vi "GeneratePSF.vi"(7 "Trans Geometry":T1={"Radius (cm)"=1.2, "a (cm)"=0.3, "focus location"=1.2} {"focus location" format="%.2f"; "a (cm)" format="%.2f"; "Radius (cm)" format="%.2f"}, 8 "Variables":T3={"Number of rings"=1, "sound spd (cm/s)"=150000, "z span (cm)"=4.0, "z steps"=20, "y spacing (cm)"=0.01, "y steps"=50, "time step (s)"=1e-08, "z"=0.0, "y"=0.0, "ref delay"=0.0, "freq (MHz)"=4.71, "cycles"=300} {"freq (MHz)" format="%.2f"; "z span (cm)" format="%.2f"; "y" format="%.2f"; "ref delay" format="%.2f"; "y spacing (cm)" format="%.2f"; "z" format="%.2f"; "time step (s)" format="%.2e"}, 9 "delay pts":i32[][](array[numeric]), 10 "h(r,t)":dbl[][][](array[numeric]) format="%.2f", 11 "Rings":T4(array[cluster]) {"focus delay abs (s)" format="%.2e"; "Waveform" format="%.2f"; "Annular rings"."a" format="%.2f"; "Annular rings"."Radius" format="%.2f"}) -> ()   [LabVIEW 2022 SP3]
uses:
  ViewData/-ReadEye/Header.ctl
  <vilib>/Analysis/2dsp.llb/Decimate (single shot, DBL).vi
  <vilib>/Analysis/baseanly.llb/Quick Scale 2D.vi
  <vilib>/Analysis/NI_AALBase.lvlib
  <vilib>/Analysis/NI_AALPro.lvlib
panel:
  in  "Resampled time step (s)":sgl=1e-09
  in  "file name":string
  in  "PSF file path":path
  in  "Header In":T2={"header info"={"Header"="", "Head length"=0}, "A/D info"={"# rf points per line"=0, "# lines per scan"=0, "sample rate MHz"=0, "# A/D bits"=0, "# bytes per A/D"=0, "TGC Flag"=0, "A/D Type"=""}, "Tranducer Info"={"bandwidth"=0.0, "center freq"=0.0, "start freq"=0.0, "ID"=0}, "Scan Info"={"delay"=0.0, "pivot distance"=0.0, "sector scan angle"=0.0, "operator"="", "Scan Mode"="", "location"=""}, "Time/Date Info"={"date"="", "time"=""}, "RF Info"={"RF file name"="", "RF file att"="", "RF cal file name"="", "RF cal file att"=""}, "Patient Info"={"ID"="", "extended ID"="", "age"=0, "sex"="", "previously\nscanned"="", "PSA"=0.0, "LOS"=1, "Ethnicty 2"=3, "Race"=3}, "Tissue Type"={"organ"=0, "disease type"=0, "disease location"=0, "IQ_pts"=0, "RcvBuffer"=0, "RcvFrame"=0, "IQBuff"=0, "IQFrame"=0, "IQPage"=0}, "Votage scaling"={"Digitizer (dB)"=0.0, "Gain (dB)"=0.0, "Atten (dB)"=0.0}, "Comment"="", "Misc Info"={"avg num"=0, "c speed"=0, "Div By or SF zones"=0, "XMIT CHS"=0, "RCV CHS"=0, "Xmit angle"=0.0}, "Therapy Parameters"={"Theraputic Freq (MHz)"=0.1, "Time on (s)"=1.0, "Therapy amplitude (mV)"=50.0, "Lines Before"=20, "Lines After"=80}, "Scan Settings"={"Energy (uJ or V)"=0, "Damp (Ohm) or Fc"=0, "HP Filt (KHz)"=0, "LP Filt (MHz)"=0, "Gain (db)"=0, "prf (kHz)"=0.0, "Distance between\nscan lines (um)"=0, "Distance between\nscan planes (um)"=0, "Scan line gap (um)"=0.0, "Scan plane gap (um)"=0.0}, "Compression Parameters"={"F1 (MHz)"=0.0, "F2 (MHz)"=0.0, "% taper"=0.0, "duration"=0.0}, "Patient Info Xtra"={"First Name"="", "Last Name"="", "Notes"=""}, "ROI Box"=[0, 0, 0, 0]} {"Compression Parameters"."% taper" min=50 max=1000 format="%.2f"; "Compression Parameters"."F2 (MHz)" format="%.3f"; "Compression Parameters"."F1 (MHz)" format="%.3f"; "Scan Settings"."prf (kHz)" format="%.2f"; "Therapy Parameters"."Therapy amplitude (mV)" min=50 max=1000 format="%.2f"; "Therapy Parameters"."Time on (s)" format="%.3f"; "Therapy Parameters"."Theraputic Freq (MHz)" format="%.3f"; "Patient Info"."Race" items=["Am Ind or Alaska", "Asian", "Hawaiian, Pac Isl", "Black or Afr Amer", "White", "more than one race", "unknown"]; "Patient Info"."Ethnicty 2" items=["Hispanic", "Non-Hispanic", "unknown"]; "Patient Info"."LOS" items=["1", "2", "3", "4", "5"]; "Patient Info"."PSA" format="%.1f"; "Scan Info"."delay" format="%.2f"; "Scan Info"."pivot distance" format="%.2f"; "Scan Info"."sector scan angle" format="%.2f"; "Tranducer Info"."bandwidth" format="%.2f"; "Tranducer Info"."center freq" format="%.2f"; "Tranducer Info"."start freq" format="%.2f"}
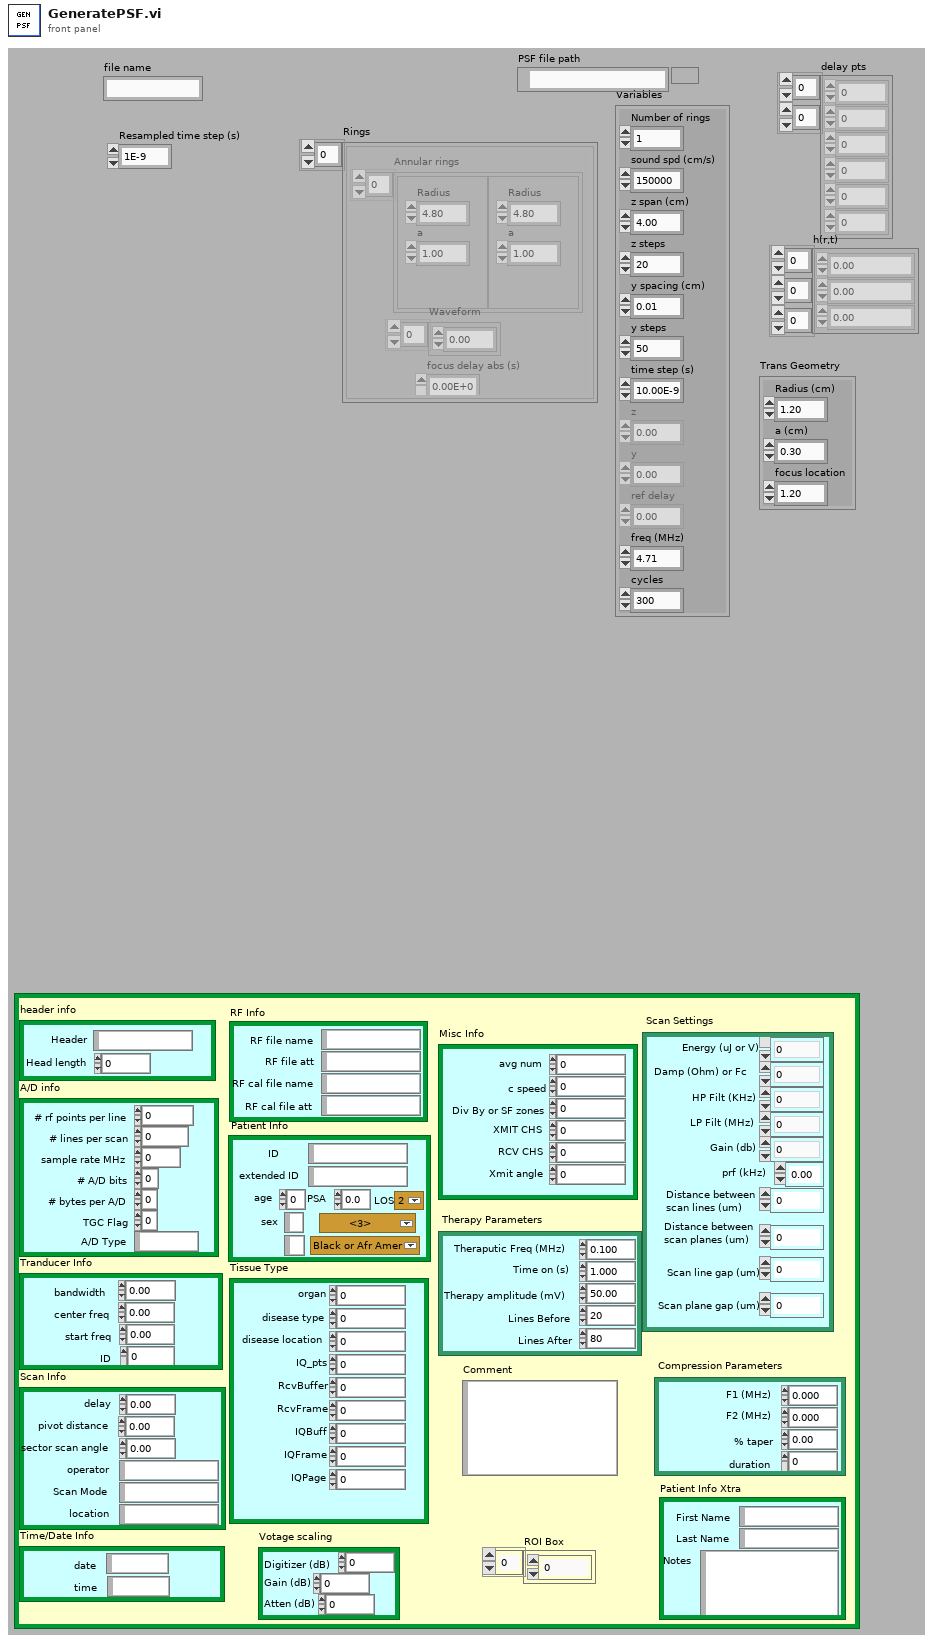
[diagram p1: front panel]
types:
  T1 = cluster{"Radius (cm)":dbl, "a (cm)":dbl, "focus location":dbl}
  T2 = typedef "Header.ctl" = cluster{"header info":cluster{"Header":string, "Head length":i16}, "A/D info":cluster{"# rf points per line":u16, "# lines per scan":u16, "sample rate MHz":u16, "# A/D bits":i16, "# bytes per A/D":u16, "TGC Flag":u16, "A/D Type":string}, "Tranducer Info":cluster{"bandwidth":sgl, "center freq":sgl, "start freq":sgl, "ID":i32}, "Scan Info":cluster{"delay":sgl, "pivot distance":sgl, "sector scan angle":sgl, "operator":string, "Scan Mode":string, "location":string}, "Time/Date Info":cluster{"date":string, "time":string}, "RF Info":cluster{"RF file name":string, "RF file att":string, "RF cal file name":string, "RF cal file att":string}, "Patient Info":cluster{"ID":string, "extended ID":string, "age":u16, "sex":string, "previously\nscanned":string, "PSA":sgl, "LOS":u8, "Ethnicty 2":u8, "Race":u8}, "Tissue Type":cluster{"organ":i16, "disease type":i16, "disease location":i16, "IQ_pts":u16, "RcvBuffer":u8, "RcvFrame":u16, "IQBuff":u8, "IQFrame":u16, "IQPage":u8}, "Votage scaling":cluster{"Digitizer (dB)":sgl, "Gain (dB)":sgl, "Atten (dB)":sgl}, "Comment":string, "Misc Info":cluster{"avg num":u16, "c speed":i16, "Div By or SF zones":i16, "XMIT CHS":u8, "RCV CHS":u8, "Xmit angle":sgl}, "Therapy Parameters":cluster{"Theraputic Freq (MHz)":sgl, "Time on (s)":sgl, "Therapy amplitude (mV)":sgl, "Lines Before":u16, "Lines After":u16}, "Scan Settings":cluster{"Energy (uJ or V)":u8, "Damp (Ohm) or Fc":u8, "HP Filt (KHz)":u8, "LP Filt (MHz)":u8, "Gain (db)":u8, "prf (kHz)":sgl, "Distance between\nscan lines (um)":u16, "Distance between\nscan planes (um)":u16, "Scan line gap (um)":sgl, "Scan plane gap (um)":sgl}, "Compression Parameters":cluster{"F1 (MHz)":sgl, "F2 (MHz)":sgl, "% taper":sgl, "duration":sgl}, "Patient Info Xtra":cluster{"First Name":string, "Last Name":string, "Notes":string}, "ROI Box":u16[]}
  T3 = cluster{"Number of rings":i32, "sound spd (cm/s)":i32, "z span (cm)":dbl, "z steps":i32, "y spacing (cm)":dbl, "y steps":i32, "time step (s)":sgl, "z":dbl, "y":dbl, "ref delay":dbl, "freq (MHz)":dbl, "cycles":i32}
  T4 = cluster{"Annular rings":cluster{"Radius":dbl, "a":dbl}[], "Waveform":dbl[], "focus delay abs (s)":dbl}[]
  T5 = cluster{"Annular rings":cluster{"Radius":dbl, "a":dbl}[], "Waveform":dbl[], "focus delay abs (s)":dbl}
  T6 = enum16{"big-endian, network order", "native, host order", "little-endian"}
  T7 = enum16{"open", "replace", "create", "open or create", "replace or create", "replace or create with confirmation"}
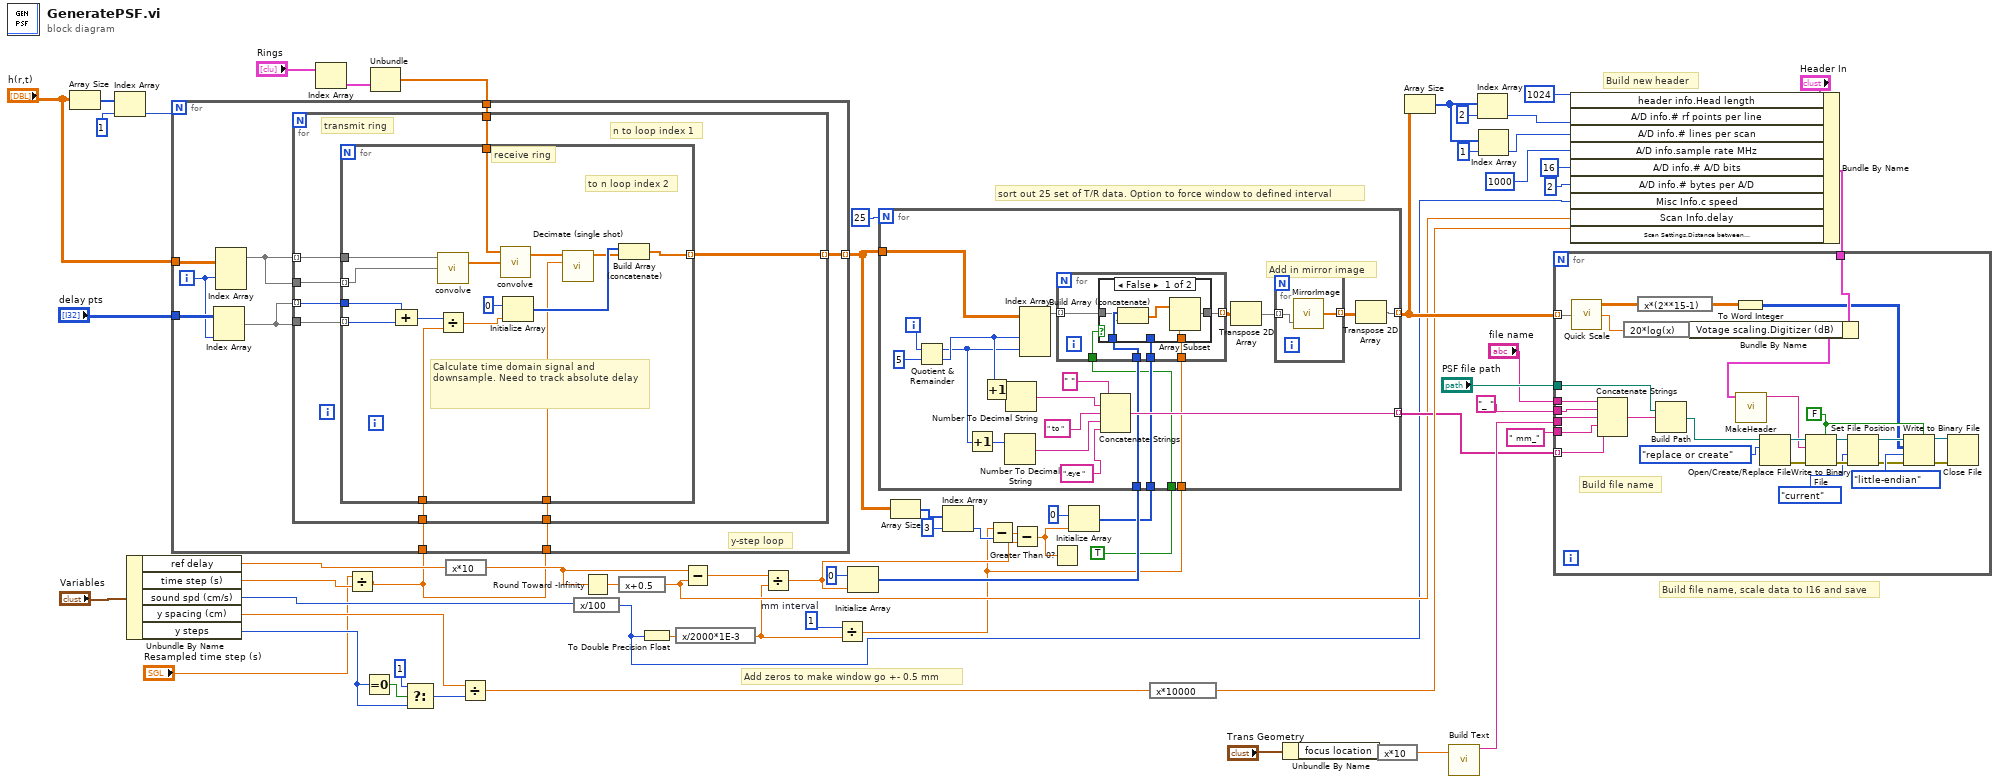
[diagram p0: block diagram]
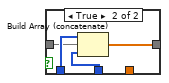
[diagram p2: hidden frame]
diagram:
  w15 = 1  # mm interval
  # "Build new header"
  # "sort out 25 set of T/R data. Option to force window to defined interval"
  # "Build file name, scale data to I16 and save"
  # "Add zeros to make window go +- 0.5 mm"
  n1 = Array Size(array="h(r,t)") -> (size(s)=w64:i32[])
  n2 = Index Array(array=w64, index=1) -> (element=w62:i32)
  n3 = Unbundle By Name("Variables") -> ("ref delay"=w42:dbl, "time step (s)"=w4:sgl, "sound spd (cm/s)"=w32:i32, "y spacing (cm)"=w37:dbl, "y steps"=w33:i32)
  n4 = Index Array(array="Rings") -> (element=w59:T5)  [unwired: 1 in]
  n5 = Divide(x="Resampled time step (s)", y=w4) -> (x/y=w3:sgl)
  n6 = Equal To 0?(x=w33) -> (x = 0?=w41:bool)
  n7 = Unbundle(w59) -> ("Waveform"=w34:dbl[])  [unwired: 2 out]
  n8 = for {
    N: w62 -> [_]
    tunnel: "h(r,t)" -> [w73]
    tunnel: "delay pts" -> [w72]
    tunnel: w34 -> [w69]
    tunnel: [w68] -> w18 mode=indexing
    tunnel: w3 -> [w67]
    tunnel: w3 -> [w65]
    i -> [w70]
    # "y-step loop"
    n9 = Index Array(array=w72, index (col)=w70) -> (element=w71:i32[])  [unwired: 1 in]
    n10 = Index Array(array=w73, index (dim 1)=w70) -> (element=w66:dbl[][])  [unwired: 2 in]
    n11 = for {
      tunnel: w66 -> [w81]
      tunnel: w66 -> [w78] mode=indexing
      tunnel: w71 -> [w80]
      tunnel: w71 -> [w79] mode=indexing
      tunnel: w69 -> [w77]
      tunnel: [w75] -> w68 mode=indexing
      tunnel: w67 -> [w76]
      tunnel: w65 -> [w74]
      # "n to loop index 1"
      # "transmit ring"
      n12 = for {
        tunnel: w78 -> [w96]
        tunnel: w81 -> [w95] mode=indexing
        tunnel: w80 -> [w93] mode=indexing
        tunnel: w79 -> [w94]
        tunnel: w77 -> [w92]
        tunnel: [w87] -> w75 mode=indexing
        tunnel: w76 -> [w90]
        tunnel: w74 -> [w82]
        # "Calculate time domain signal and downsample. Need to track absolute delay"
        # "to n loop index 2"
        # "receive ring"
        n13 = Compound Arithmetic op=ADD(w94, w93) -> (w91:i32)
        n14 = call "convolve.vi"("X"=w96, "Y"=w95) -> ("X*Y"=w85:dbl[])  [unwired: 2 in, 2 out]
        n15 = Divide(x=w91, y=w90) -> (x/y=w88:sgl)
        n16 = call "convolve.vi"("X"=w92, "Y"=w85) -> ("X*Y"=w84:dbl[])  [unwired: 2 in, 2 out]
        n17 = Initialize Array(i16 0, w88) -> (w86:i16[])
        n18 = call-poly <vilib>:"Decimate (single shot).vi"("decimating factor"=w82, "X"=w84) -> ("Decimated Array"=w83:dbl[])  [unwired: 8 in, 1 out]
        n19 = Build Array (concatenate)(w86, w83) -> (w87:dbl[])
      }
    }
  }
  n20 = Select(t=1, s=w41, f=w33) -> (s? t:f=w40:i32)
  n21 = expression code="x*10"(w42) -> (w23:dbl)
  n22 = Divide(x=w37, y=w40) -> (x/y=w36:dbl)
  n23 = expression code="x/100"(w32) -> (w1:i32)
  n24 = Round Toward -Infinity(1:w23) -> (0:w24:dbl)
  n25 = expression code="x+0.5"(w24) -> (w17:dbl)
  n26 = To Double Precision Float(number=w1) -> (double precision float=w22:dbl)
  n27 = expression code="x/2000*1E-3"(w22) -> (w16:dbl)
  n28 = Subtract(x=w23, y=w17) -> (x-y=w21:dbl)
  n29 = Divide(x=w21, y=w16) -> (x/y=w8:dbl)
  n30 = Divide(x=w15, y=w16) -> (x/y=w6:dbl)
  n31 = Initialize Array(i16 0, w8) -> (w19:i16[])
  n32 = Array Size(array=w18) -> (size(s)=w14:i32[])
  n33 = Index Array(array=w14, index=3) -> (element=w10:i32)
  n34 = Subtract(x=w6, y=w10) -> (x-y=w9:dbl)
  n35 = Subtract(x=w9, y=w8) -> (x-y=w7:dbl)
  n36 = Greater Than 0?(x=w7) -> ()  [unwired: 1 out]
  n37 = Initialize Array(i16 0, w7) -> (w11:i16[])
  n38 = for {
    N: 25 -> [_]
    tunnel: w18 -> [w118]
    tunnel: [w103] -> w43 mode=indexing
    tunnel: [w112] -> w26 mode=indexing
    tunnel: w19 -> [w101]
    tunnel: w11 -> [w100]
    tunnel: TRUE -> [w98]
    tunnel: w6 -> [w97]
    i -> [w117]
    # "Add in mirror image"
    n39 = Quotient & Remainder(x=w117, y=5) -> (x-y*floor(x/y)=w114:i32, floor(x/y)=w115:i32)
    n40 = Increment(x=w114) -> (x+1=w108:i32)
    n41 = Increment(x=w115) -> (x+1=w109:i32)
    n42 = Number To Decimal String(number=w108) -> (decimal integer string=w113:string)  [unwired: 1 in]
    n43 = Number To Decimal String(number=w109) -> (decimal integer string=w110:string)  [unwired: 1 in]
    n44 = Index Array(array=w118, index (dim 1)=w115, index (dim 2)=w114) -> (element=w102:dbl[][])  [unwired: 2 in]
    n45 = for {
      tunnel: w102 -> [w123] mode=indexing
      tunnel: w101 -> [w124]
      tunnel: w100 -> [w122]
      tunnel: [w121] -> w99 mode=indexing
      tunnel: w98 -> [w120]
      tunnel: w97 -> [w119]
      n46 = case shown="False" w120 {
        tunnel: w124 -> [w129 w133]
        tunnel: w123 -> [w128 w132]
        tunnel: w122 -> [_ w131]
        tunnel: [w126 w130] -> w121
        tunnel: w119 -> [w125 _]
        frame False {
          n47 = Build Array (concatenate)(w129, w128) -> (w127:dbl[])
          n48 = Array Subset(array=w127, length=w125) -> (w126:dbl[])  [unwired: 1 in]
        }
        frame True {
          n49 = Build Array (concatenate)(w133, w132, w131) -> (w130:dbl[])
        }
      }
    }
    n50 = Concatenate Strings(" ", w110, " to ", w113, ".eye ") -> (w112:string)
    n51 = Transpose 2D Array(2D array=w99) -> (transposed array=w106:dbl[][])
    n52 = for {
      tunnel: w106 -> [w135] mode=indexing
      tunnel: [w134] -> w107 mode=indexing
      n53 = call "MirrorImage.vi"("input"=w135) -> ("output"=w134:dbl[])  [unwired: 1 in, 1 out]
    }
    n54 = Transpose 2D Array(2D array=w107) -> (transposed array=w103:dbl[][])
  }
  n55 = expression code="x*10000"(w36) -> (w35:dbl)
  n56 = Unbundle By Name("Trans Geometry") -> ("focus location"=w30:dbl)
  n57 = expression code="x*10"(w30) -> (w25:dbl)
  n58 = Array Size(array=w43) -> (size(s)=w52:i32[])
  n59 = call "Build Text"("d"=w25) -> ("Result"=w28:string)  [unwired: 13 in, 1 out]
  n60 = Index Array(array=w52, index=2) -> (element=w54:i32)
  n61 = Index Array(array=w52, index=1) -> (element=w51:i32)
  n62 = Bundle By Name(cluster="Header In", "header info.Head length"=i16 1024, "A/D info.# rf points per line"=w54, "A/D info.# lines per scan"=w51, "A/D info.sample rate MHz"=u16 1000, "A/D info.# A/D bits"=i16 16, "A/D info.# bytes per A/D"=u16 2, "Misc Info.c speed"=w1, "Scan Info.delay"=w17, "Scan Settings.Distance between\nscan lines (um)"=w35) -> (w48:T2)
  n63 = for {
    tunnel: w43 -> [w151] mode=indexing
    tunnel: w48 -> [w149]
    tunnel: "PSF file path" -> [w145]
    tunnel: w26 -> [w137] mode=indexing
    tunnel: "file name" -> [w140]
    tunnel: "_ " -> [w139]
    tunnel: w28 -> [w138]
    tunnel: " mm_" -> [w136]
    w163 = FALSE ("prepend array or string size? (T)")
    # "Build file name"
    n64 = call-poly <vilib>:"Quick Scale.vi"("X"=w151) -> ("Yij=Xij/Max|X|"=w142:dbl[][], "max|X|"=w147:dbl)  [unwired: 1 out]
    n65 = Concatenate Strings(w140, w139, w138, w136, w137) -> (w144:string)
    n66 = expression code="20*log(x)"(w147) -> (w148:dbl)
    n67 = expression code="x*(2**15-1)"(w142) -> (w150:dbl[][])
    n68 = Build Path(base path=w145, name or relative path=w144) -> (appended path=w143:path)
    n69 = Bundle By Name(cluster=w149, "Votage scaling.Digitizer (dB)"=w148) -> (w146:T2)
    n70 = To Word Integer(number=w150) -> (16bit integer=w141:i16[][])
    n71 = call "MakeHeader.vi"("Header In"=w146) -> ("Header String"=w152:string)  [unwired: 6 out]
    n72 = Open/Create/Replace File(file path (use dialog)=w143, operation (0:open)=T7."replace or create") -> (refnum out=w159:refnum<file>, error out=w160:errorcluster)  [unwired: 1 in, 4 out]
    n73 = Write to Binary File(file (use dialog)=w159, data=w152, error in=w160, 5:w163) -> (refnum out=w157:refnum<file>, error out=w158:errorcluster)  [unwired: 3 out]
    n74 = Set File Position(refnum=w157, from (0:start)=enum16{"start", "end", "current"}."current" ("pos mode (0:2)"), error in=w158) -> (refnum out=w161:refnum<file>, error out=w162:errorcluster)  [unwired: 1 out]
    n75 = Write to Binary File(file (use dialog)=w161, data=w141, error in=w162, 5:w163, 9:T6."little-endian" ("byte order (0:big-endian, network order)")) -> (refnum out=w155:refnum<file>, error out=w154:errorcluster)  [unwired: 2 out]
    n76 = Close File(refnum=w155, error in=w154) -> ()  [unwired: 2 out]
  }
